vi "Hangup Test.vi"(6 "Aktion Hangup Test":T1, 8 "Status":string, 9 "FID":sgl caption="ppm" format="%.1f") -> (0 "Status":string, 1 "Test beendet?":bool, 2 "countdonw":dbl, 4 "Aktion Hangup Test 2":T1)   [LabVIEW 2020, in "Hangup Check.lvlib"]
uses:
  Hangup Check.lvlib
  Aktion Hangup Test.ctl
  Amium PNS/Aktion FGV Amium Daten.ctl
  AktionFGV Hangup.ctl
  Seiten/CalGas Aufschaltung/FGV CalGas Aktionen.ctl
  Seiten/CalGas Aufschaltung/Auswahl Analysator.ctl
  Analysator Definition/FGV Analysator Definition Aktionen.ctl
  Sprachverwaltung/FGV Aktion Tabelle zerlegen.ctl
  Funktionstasten/Funktionstasten-Aktion.ctl
  Funktionstasten/Zustaende.ctl
  Messdaten/Gewichtung (Stichprobe).ctl
  Seiten/CalGas Aufschaltung/CalGas Aufschaltung.lvlib
  Seiten/FT-IR/FT-IR.lvlib
  Sprachverwaltung/Sprachverwaltung.lvlib
  Funktionstasten/Funktionstasten.lvlib
  Analysator Definition/Analysator Definition.lvlib
  Seiten/FT-IR/FGV FT-IR Aktionen.ctl
  Messdaten/Messdaten.lvlib
  Messdaten/Aktionen FGV Messdaten.ctl
  Amium PNS/Amium PNS.lvlib
  Linearisierung V2/Linearisierung v2.lvlib
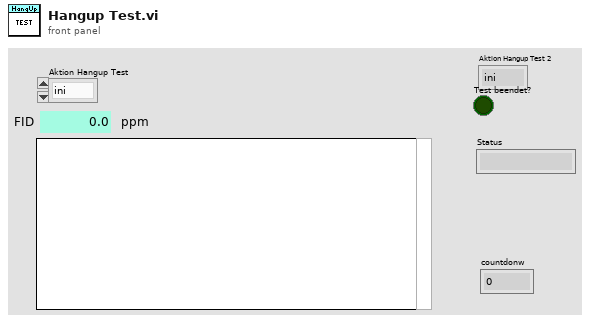
[diagram p1: front panel]
types:
  T1 = typedef "Hangup Check.lvlib/Aktion Hangup Test.ctl" = enum16{"ini", "0-Gas aufschalten", "warten", "E-Gas aufschalten", "auswerten", "Fertig"}
  T2 = typedef "Amium PNS.lvlib/Aktion FGV Amium Daten.ctl" = enum16{"lesen", "Komm Daten", "Daten", "Error", "Regler", "Grenzwerte", "laden", "speichern"}
  T3 = typedef "Sprachverwaltung.lvlib/FGV Aktion Tabelle zerlegen.ctl" = enum16{"laden", "vereinzeln", "speichern"}
  T4 = typedef "Analysator Definition.lvlib/FGV Analysator Definition Aktionen.ctl" = enum16{"lesen", "MB setzen", "MB KAL setzen", "laden"}
  T5 = typedef "CalGas Aufschaltung.lvlib/Auswahl Analysator.ctl" = enum16{"FT-IR", "FID", "PMA", "PMA/FID/FT-IR"}
  T6 = typedef "CalGas Aufschaltung.lvlib/FGV CalGas Aktionen.ctl" = enum16{"lesen", "Analysator Auswahl", "Def.CalGas", "Aufschaltung CalGas", "laden", "speichern", "KAL extrahieren"}
  T7 = typedef "Hangup Check.lvlib/AktionFGV Hangup.ctl" = enum16{"lesen", "Hangup Settings", "Protokoll", "Pfad", "laden", "speichern"}
  T8 = typedef "Funktionstasten.lvlib/Zustaende.ctl" = enum16{"Standby", "Pause", "Eco", "Messen", "Kalibrieren", "Spülen Filter", "Spülen Leitung", "Umgebungsluft", "0-Gas", "Cal-Gas", "CG zu PNS", "-------------", "Init 1", "Init 2", "Init 3", "Init 4", "Messen vorbereiten", "Messen durchführen", "Exit"}
  T9 = typedef "Funktionstasten.lvlib/Funktionstasten-Aktion.ctl" = enum16{"Initialisieren", "Zustand setzen", "Taste gedrückt", "Fehler speichern", "Lesen", "Manuell", "Remote", "Bitparallel", "Samplepoint", "Zeit Prüfen", "reset Umschalten"}
  T10 = typedef "Messdaten.lvlib/Aktionen FGV Messdaten.ctl" = enum16{"lesen", "schreiben", "löschen", "Mittelwerte", "Komponente"}
  T11 = typedef "Messdaten.lvlib/Gewichtung (Stichprobe).ctl" = enum16{"Sample", "Population"}
  T12 = typedef "FT-IR.lvlib/FGV FT-IR Aktionen.ctl" = enum16{"lesen", "NOG setzen", "NOS setzen", "Initialisieren", "speichern", "ALLES setzen", "FT-IR Spektrum loggen", "Komm Stoppen", "Spektrum LogKonfig"}
  T13 = typedef "Amium PNS.lvlib/Daten Cluster.ctl" = cluster{"Amium Zustände":T14, "Samplepoint am PNS":i16, "Gerätekennung":string, "aktiver Samplepoint":i16[], "Messgasdruck":sgl}
  T14 = typedef "Amium PNS.lvlib/Amium Zustand.ctl" = u16
  T15 = typedef "Hangup Check.lvlib/HangupSettings.ctl" = cluster{"Kalibriergas":T16, "Aufschaltpunkt":T16, "Spangas Aufschaltzeit:":sgl, "Nullgas Aufschaltzeit:":sgl, "Datenerfassungszeit:":sgl, "Grenzwert manuell:":sgl, "Grenzwert:":sgl, "Grenze":T16, "Messbereich":T16, "Spankonzentration [ppm]":sgl, "Grenzwert: C1":sgl}
  T16 = typedef "Auswahlfeld.ctl" = u16
  T17 = typedef "Analysator Definition.lvlib/Betriebsdaten Komponente.ctl" = cluster{"Namen":string[], "MB Namen":string[], "Einheit":string, "MB Aktuell":u16, "MB Endwert":u16, "CalGase":u16[], "MB für KAL":u16[], "CG für KAL":u16[]}
  T18 = typedef "CalGas Aufschaltung.lvlib/Aufschaltung CalGas.ctl" = cluster{"Kalibriergas":T16, "Aufschaltpunkt":T19, "Analysator":T5}
  T19 = typedef "CalGas Aufschaltung.lvlib/Auswahl Aufschaltpunkt.ctl" = enum16{"über Filterblock", "Analysator direkt", "über PNS", "Entnahme", "Gasdivider"}
  T20 = typedef "Zahlen-Eingabefeld.ctl" = sgl
  T21 = typedef "Hangup Check.lvlib/Protokoll.ctl" = cluster{"FID Mittelwert 0":sgl, "FID Mittelwert E":sgl, "Messgasdruck Amium":sgl, "Startzeit":timestamp, "Endzeit":timestamp, "Bestanden?":bool}
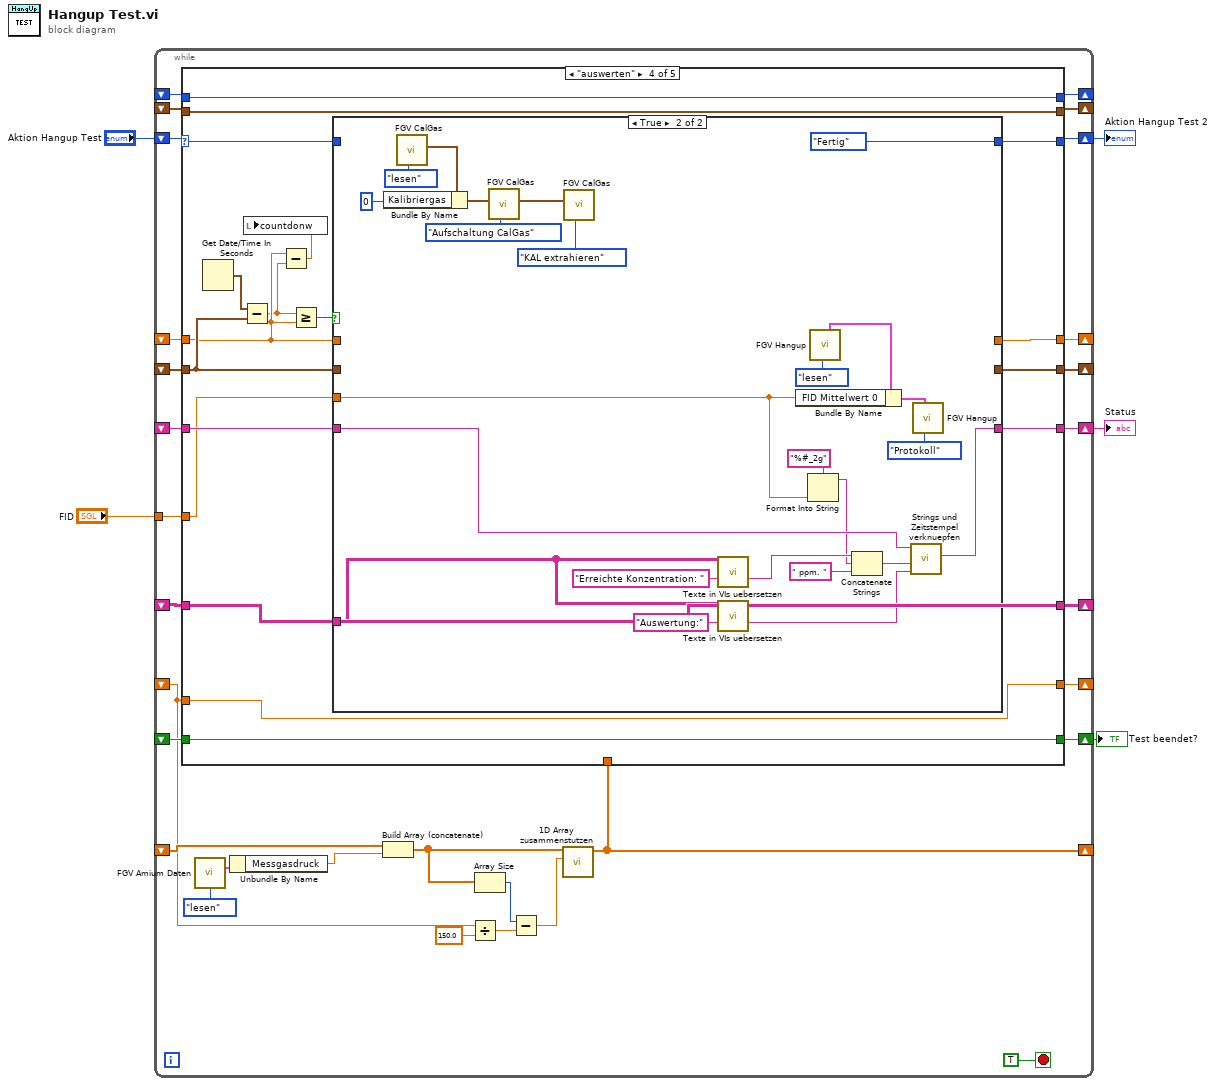
[diagram p0: block diagram]
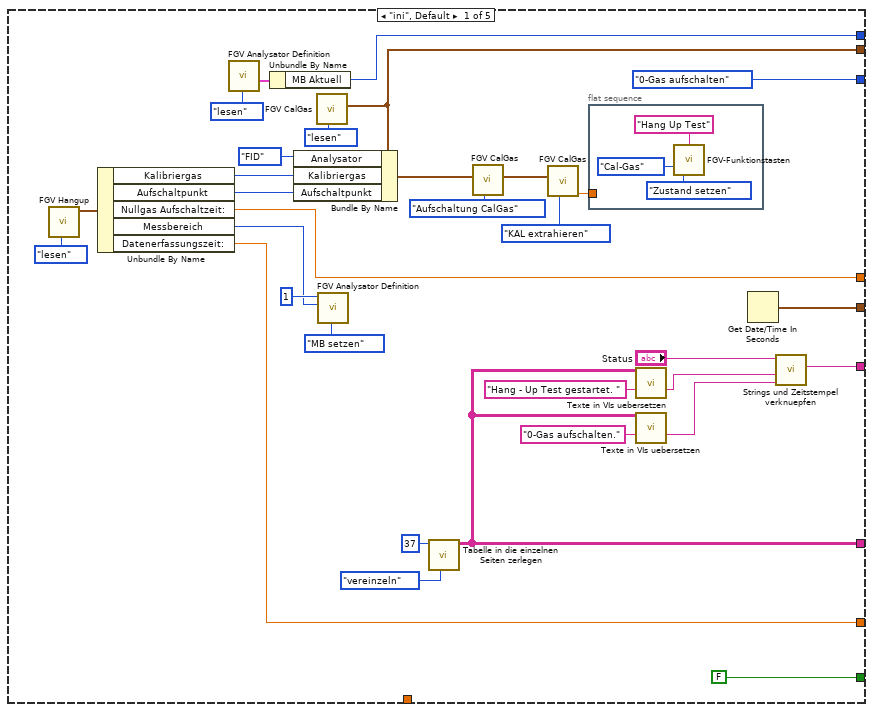
[diagram p2: hidden frame]
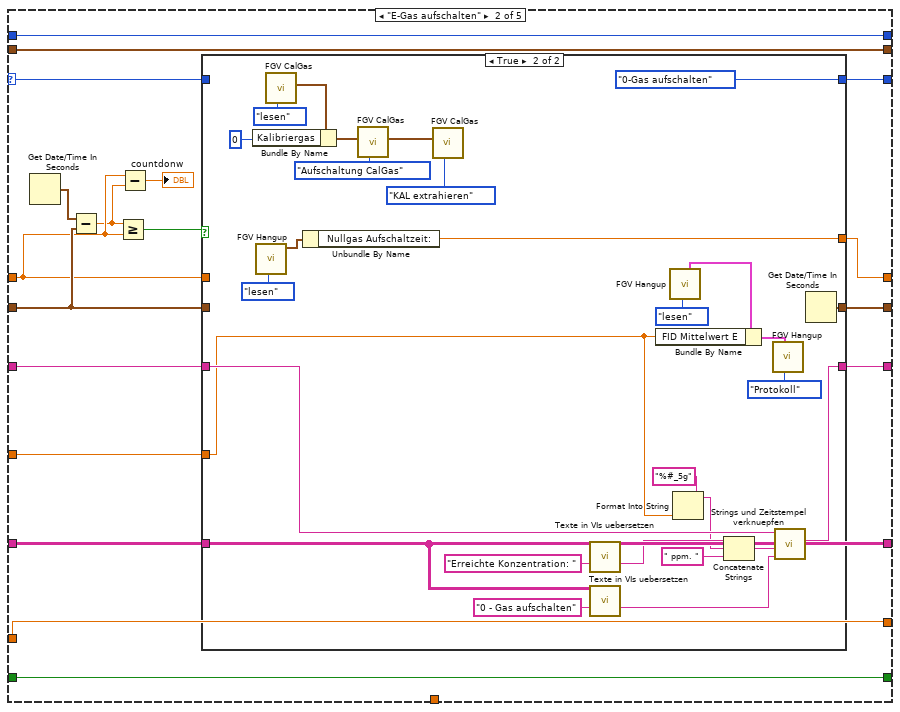
[diagram p3: hidden frame]
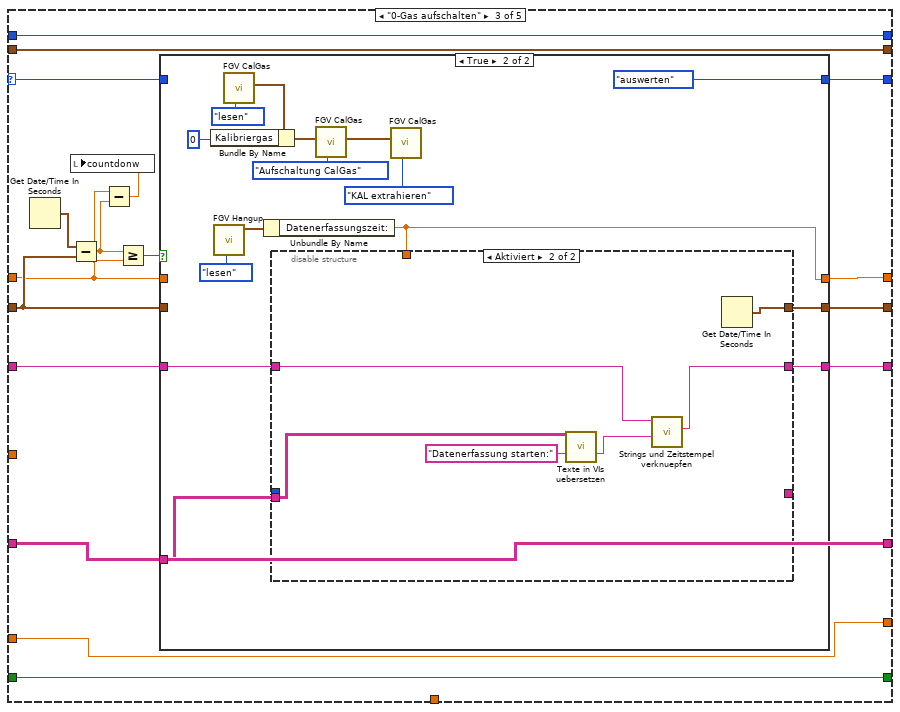
[diagram p5: hidden frame]
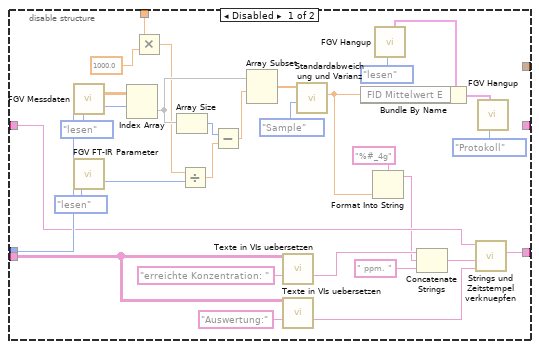
[diagram p7: hidden frame]
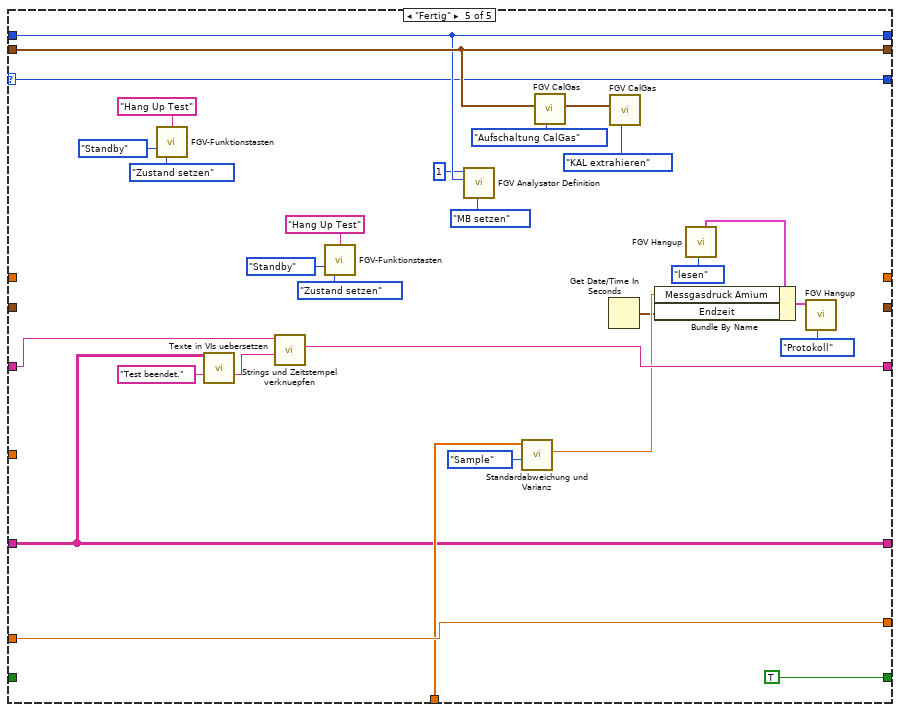
[diagram p9: hidden frame]
diagram:
  n1 = while {
    shift-right: [w34] -> _
    shift-left: _ -> [w33]
    shift-right: [w32] -> w4
    shift-left: _ -> [w31]
    shift-right: [w30] -> _
    shift-left: _ -> [w29]
    shift-right: [w28] -> _
    shift-left: _ -> [w27]
    shift-right: [w26] -> w3
    shift-left: "Aktion Hangup Test" -> [w25]
    shift-right: [w24] -> _
    shift-left: _ -> [w23]
    shift-right: [w22] -> w2
    shift-left: _ -> [w21]
    shift-right: [w9] -> _
    shift-left: _ -> [w18]
    shift-right: [w11] -> _
    shift-left: _ -> [w10]
    shift-right: [w8] -> _
    shift-left: _ -> [w7]
    tunnel: "FID" -> [w6]
    stop <- TRUE stop-if-true
    n2 = call "FGV Amium Daten.vi"("Aktion"=Aktion_FGV_Amium_Daten."lesen") -> ("Amium Daten"=w20:T13)  [unwired: 9 in, 5 out]
    n3 = Unbundle By Name(w20) -> ("Messgasdruck"=w17:sgl)
    n4 = Build Array (concatenate)(w18, w17) -> (w14:sgl[])
    n5 = Divide(x=w10, y=sgl 150.0) -> (x/y=w15:sgl)
    n6 = Array Size(array=w14) -> (size(s)=w16:i32)
    n7 = Subtract(x=w16, y=w15) -> (x-y=w12:sgl)
    n8 = call "1D Array zusammenstutzen.vi"("Anzahl Elemente"=w12, "Messdaten"=w14) -> ("Messdaten"=w9:sgl[])  [unwired: 8 in, 1 out]
    n9 = case shown="\"auswerten\"" w25 {
      selector: w25 -> [_ w85 w134 w207 w250]
      tunnel: [w58 w88 w137 w210 w263] -> w34
      tunnel: w33 -> [_ w88 w137 w210 w263]
      tunnel: [w54 w81 w130 w203 w251] -> w32
      tunnel: w31 -> [_ w82 w131 w204 w252]
      tunnel: [w50 w79 w128 w201 _] -> w30
      tunnel: w29 -> [_ w78 w129 w202 _]
      tunnel: [w49 w80 w127 w200 _] -> w28
      tunnel: w27 -> [_ w74 w123 w196 _]
      tunnel: [Aktion_Hangup_Test."0-Gas aufschalten" ("Aktion Hangup Test") w84 w133 w206 w250] -> w26
      tunnel: [w42 w83 w132 w205 w261] -> w24
      tunnel: w23 -> [_ w83 w132 w205 w261]
      tunnel: [FALSE w77 w126 w199 TRUE] -> w22
      tunnel: w21 -> [_ w77 w126 w199 _]
      tunnel: [w39 w76 w125 w198 w256] -> w11
      tunnel: w10 -> [_ w76 w125 w198 w256]
      tunnel: w9 -> [_ _ _ _ w255]
      tunnel: [w36 w75 w124 w197 w249] -> w8
      tunnel: w7 -> [_ w75 w124 w197 w249]
      tunnel: w6 -> [_ w71 _ w193 _]
      frame "ini", Default {
        n10 = call "FGV Hangup.vi"("Aktion"=AktionFGV_Hangup."lesen") -> ("Hangup Settings"=w66:T15)  [unwired: 6 in, 4 out]
        n11 = Unbundle By Name(w66) -> ("Kalibriergas"=w51:T16, "Aufschaltpunkt"=w59:T16, "Nullgas Aufschaltzeit:"=w49:sgl, "Messbereich"=w41:T16, "Datenerfassungszeit:"=w39:sgl)
        n12 = call "FGV Analysator Definition.vi"("Aktionen"=FGV_Analysator_Definition_Aktionen."lesen") -> ("Betriebsdaten Komponente"=w43:T17)  [unwired: 6 in, 4 out]
        n13 = Unbundle By Name(w43) -> ("MB Aktuell"=w42:u16)
        n14 = call "FGV CalGas.vi"("Aktionen"=FGV_CalGas_Aktionen."lesen") -> ("Aufschaltung CalGas"=w58:T18)  [unwired: 6 in, 4 out]
        n15 = Bundle By Name(cluster=w58, "Analysator"=Auswahl_Analysator."FID", "Kalibriergas"=w51, "Aufschaltpunkt"=w59) -> (w65:T18)
        n16 = call "FGV Analysator Definition.vi"("Aktionen"=FGV_Analysator_Definition_Aktionen."MB setzen", "Messbereich"=w41, "Komponente"=1) -> ()  [unwired: 4 in, 5 out]
        n17 = call "Tabelle in die einzelnen Seiten zerlegen.vi"("Aktion"=FGV_Aktion_Tabelle_zerlegen."vereinzeln", "Index (Seite)"=37) -> ("Sprachliste"=w36:string[][])  [unwired: 7 in, 2 out]
        n18 = call "FGV CalGas.vi"("Aktionen"=FGV_CalGas_Aktionen."Aufschaltung CalGas", "Aufschaltung CalGas"=w65) -> ("Aufschaltung CalGas"=w62:T18)  [unwired: 5 in, 4 out]
        n19 = call "FGV CalGas.vi"("Aktionen"=FGV_CalGas_Aktionen."KAL extrahieren", "Aufschaltung CalGas"=w62) -> ("Konzentration 2"=w48:T20)  [unwired: 5 in, 4 out]
        n20 = flat-sequence {
          tunnel: w48 -> [_]
          frame #0 {
            n21 = call "FGV-Funktionstasten.vi"("Herkunft"="Hang Up Test", "Zustand"=Zustaende."Cal-Gas", "Aktion"=Funktionstasten-Aktion."Zustand setzen") -> ()  [unwired: 5 in, 8 out]
          }
        }
        n22 = call "Texte in VIs uebersetzen.vi"("Sprachliste"=w36, "String zum Übersetzen"="Hang - Up Test gestartet. ") -> ("String zum Übersetzen"=w56:string)  [unwired: 9 in, 4 out]
        n23 = call "Texte in VIs uebersetzen.vi"("Sprachliste"=w36, "String zum Übersetzen"="0-Gas aufschalten.") -> ("String zum Übersetzen"=w53:string)  [unwired: 9 in, 4 out]
        n24 = Get Date/Time In Seconds() -> (seconds since 1Jan1904=w50:timestamp)
        n25 = call "Strings und Zeitstempel verknuepfen.vi"("String 2 hinzufügen"=w53, "String 1 hinzufügen"=w56, "Eingagns String"="Status") -> ("Verknüpfter String"=w54:string)  [unwired: 8 in]
      }
      frame "E-Gas aufschalten" {
        n26 = Get Date/Time In Seconds() -> (seconds since 1Jan1904=w87:timestamp)
        n27 = Subtract(x=w87, y=w78) -> (x-y=w73:dbl)
        n28 = Greater Or Equal?(x=w73, y=w74) -> (x >= y?=w86:bool)
        n29 = Subtract(x=w74, y=w73) -> (x-y=→"countdonw":dbl)
        n30 = case shown="True" w86 {
          tunnel: w85 -> [w92 _]
          tunnel: [w92 Aktion_Hangup_Test."0-Gas aufschalten" ("Aktion Hangup Test")] -> w84
          tunnel: w82 -> [w91 w109]
          tunnel: [w91 w108] -> w81
          tunnel: [w89 w107] -> w80
          tunnel: [w90 w106] -> w79
          tunnel: w78 -> [w90 _]
          tunnel: w74 -> [w89 _]
          tunnel: w75 -> [_ w98]
          tunnel: w71 -> [_ w93]
          frame False {
          }
          frame True {
            n31 = call "FGV Hangup.vi"("Aktion"=AktionFGV_Hangup."lesen") -> ("Hangup Settings"=w112:T15)  [unwired: 6 in, 4 out]
            n32 = call "FGV CalGas.vi"("Aktionen"=FGV_CalGas_Aktionen."lesen") -> ("Aufschaltung CalGas"=w114:T18)  [unwired: 6 in, 4 out]
            n33 = Bundle By Name(cluster=w114, "Kalibriergas"=0) -> (w119:T18)
            n34 = Unbundle By Name(w112) -> ("Nullgas Aufschaltzeit:"=w107:sgl)
            n35 = call "FGV CalGas.vi"("Aktionen"=FGV_CalGas_Aktionen."Aufschaltung CalGas", "Aufschaltung CalGas"=w119) -> ("Aufschaltung CalGas"=w116:T18)  [unwired: 5 in, 4 out]
            n36 = call "FGV CalGas.vi"("Aktionen"=FGV_CalGas_Aktionen."KAL extrahieren", "Aufschaltung CalGas"=w116) -> ()  [unwired: 5 in, 5 out]
            n37 = call "Texte in VIs uebersetzen.vi"("Sprachliste"=w98, "String zum Übersetzen"="Erreichte Konzentration: ") -> ("String zum Übersetzen"=w102:string)  [unwired: 9 in, 4 out]
            n38 = call "Texte in VIs uebersetzen.vi"("Sprachliste"=w98, "String zum Übersetzen"="0 - Gas aufschalten") -> ("String zum Übersetzen"=w104:string)  [unwired: 9 in, 4 out]
            n39 = call "FGV Hangup.vi"("Aktion"=AktionFGV_Hangup."lesen") -> ("Protokoll"=w95:T21)  [unwired: 6 in, 4 out]
            n40 = Bundle By Name(cluster=w95, "FID Mittelwert E"=w93) -> (w97:T21)
            n41 = Format Into String(format string="%#_5g" ("Format-String"), w93) -> (resulting string=w101:string)  [unwired: 2 in, 1 out]
            n42 = Concatenate Strings(w102, w101, " ppm. " ("String")) -> (w99:string)
            n43 = call "FGV Hangup.vi"("Aktion"=AktionFGV_Hangup."Protokoll", "Protokoll"=w97) -> ()  [unwired: 5 in, 5 out]
            n44 = call "Strings und Zeitstempel verknuepfen.vi"("String 2 hinzufügen"=w104, "String 1 hinzufügen"=w99, "Eingagns String"=w109) -> ("Verknüpfter String"=w108:string)  [unwired: 8 in]
            n45 = Get Date/Time In Seconds() -> (seconds since 1Jan1904=w106:timestamp)
          }
        }
      }
      frame "0-Gas aufschalten" {
        n46 = Get Date/Time In Seconds() -> (seconds since 1Jan1904=w136:timestamp)
        n47 = Subtract(x=w136, y=w129) -> (x-y=w122:dbl)
        n48 = Subtract(x=w123, y=w122) -> (x-y=w121:dbl)
        n49 = local write "countdonw"(w121) -> ()
        n50 = Greater Or Equal?(x=w122, y=w123) -> (x >= y?=w135:bool)
        n51 = case shown="True" w135 {
          tunnel: w134 -> [w141 _]
          tunnel: [w141 Aktion_Hangup_Test."auswerten" ("Aktion Hangup Test")] -> w133
          tunnel: w131 -> [w140 w146]
          tunnel: [w140 w143] -> w130
          tunnel: w129 -> [w139 _]
          tunnel: [w139 w142] -> w128
          tunnel: [w138 w144] -> w127
          tunnel: w123 -> [w138 _]
          tunnel: w124 -> [_ w145]
          frame False {
          }
          frame True {
            n52 = call "FGV Hangup.vi"("Aktion"=AktionFGV_Hangup."lesen") -> ("Hangup Settings"=w148:T15)  [unwired: 6 in, 4 out]
            n53 = call "FGV CalGas.vi"("Aktionen"=FGV_CalGas_Aktionen."lesen") -> ("Aufschaltung CalGas"=w150:T18)  [unwired: 6 in, 4 out]
            n54 = Bundle By Name(cluster=w150, "Kalibriergas"=0) -> (w155:T18)
            n55 = Unbundle By Name(w148) -> ("Datenerfassungszeit:"=w144:sgl)
            n56 = disable-structure shown="Aktiviert" {
              disable-tunnel: _ -> [w174 _]
              disable-tunnel: [w169 _] -> _
              disable-tunnel: w146 -> [w168 w191]
              disable-tunnel: w145 -> [w163 w188]
              disable-tunnel: w144 -> [w157 _]
              disable-tunnel: [_ w190] -> w143
              disable-tunnel: [_ w187] -> w142
              frame Disabled {
                n57 = call "FGV Messdaten.vi"("Aktionen"=Aktionen_FGV_Messdaten."lesen") -> ("Messdaten"=w177:sgl[][])  [unwired: 6 in, 8 out]
                n58 = call "FGV FT-IR Parameter.vi"("Aktion"=FGV_FT-IR_Aktionen."lesen") -> ("Zykluszeit Messdatenverteiler"=w186:u32)  [unwired: 11 in, 7 out]
                n59 = Index Array(array=w177, index (row)=w174) -> (element=w178:sgl[])  [unwired: 1 in]
                n60 = Multiply(x=w157, y=sgl 1000.0) -> (x*y=w175:sgl)
                n61 = Array Size(array=w178) -> (size(s)=w181:i32)
                n62 = Divide(x=w175, y=w186) -> (x/y=w180:sgl)
                n63 = Subtract(x=w181, y=w180) -> (x-y=w182:sgl)
                n64 = Array Subset(array=w178, index=w182) -> (w179:sgl[])  [unwired: 1 in]
                n65 = call "Texte in VIs uebersetzen.vi"("Sprachliste"=w163, "String zum Übersetzen"="erreichte Konzentration: ") -> ("String zum Übersetzen"=w172:string)  [unwired: 9 in, 4 out]
                n66 = call "Texte in VIs uebersetzen.vi"("Sprachliste"=w163, "String zum Übersetzen"="Auswertung:") -> ("String zum Übersetzen"=w173:string)  [unwired: 9 in, 4 out]
                n67 = call "Standardabweichung und Varianz.vi"("Gewichtung (Stichprobe)"=Gewichtung_(Stichprobe)."Sample", "X"=w179) -> ("Mittelwert"=w158:sgl)  [unwired: 7 in, 2 out]
                n68 = Format Into String(format string="%#_4g" ("Format-String"), w158) -> (resulting string=w164:string)  [unwired: 2 in, 1 out]
                n69 = call "FGV Hangup.vi"("Aktion"=AktionFGV_Hangup."lesen") -> ("Protokoll"=w160:T21)  [unwired: 6 in, 4 out]
                n70 = Bundle By Name(cluster=w160, "FID Mittelwert E"=w158) -> (w162:T21)
                n71 = Concatenate Strings(w172, w164, " ppm. " ("String")) -> (w170:string)
                n72 = call "Strings und Zeitstempel verknuepfen.vi"("String 2 hinzufügen"=w173, "String 1 hinzufügen"=w170, "Eingagns String"=w168) -> ("Verknüpfter String"=w169:string)  [unwired: 8 in]
                n73 = call "FGV Hangup.vi"("Aktion"=AktionFGV_Hangup."Protokoll", "Protokoll"=w162) -> ()  [unwired: 5 in, 5 out]
              }
              frame Enabled {
                n74 = call "Texte in VIs uebersetzen.vi"("Sprachliste"=w188, "String zum Übersetzen"="Datenerfassung starten:") -> ("String zum Übersetzen"=w189:string)  [unwired: 9 in, 4 out]
                n75 = call "Strings und Zeitstempel verknuepfen.vi"("String 1 hinzufügen"=w189, "Eingagns String"=w191) -> ("Verknüpfter String"=w190:string)  [unwired: 9 in]
                n76 = Get Date/Time In Seconds() -> (seconds since 1Jan1904=w187:timestamp)
              }
            }
            n77 = call "FGV CalGas.vi"("Aktionen"=FGV_CalGas_Aktionen."Aufschaltung CalGas", "Aufschaltung CalGas"=w155) -> ("Aufschaltung CalGas"=w152:T18)  [unwired: 5 in, 4 out]
            n78 = call "FGV CalGas.vi"("Aktionen"=FGV_CalGas_Aktionen."KAL extrahieren", "Aufschaltung CalGas"=w152) -> ()  [unwired: 5 in, 5 out]
          }
        }
      }
      frame "auswerten" {
        n79 = Get Date/Time In Seconds() -> (seconds since 1Jan1904=w209:timestamp)
        n80 = Subtract(x=w209, y=w202) -> (x-y=w195:dbl)
        n81 = Subtract(x=w196, y=w195) -> (x-y=w194:dbl)
        n82 = local write "countdonw"(w194) -> ()
        n83 = Greater Or Equal?(x=w195, y=w196) -> (x >= y?=w208:bool)
        n84 = case shown="True" w208 {
          tunnel: w207 -> [w214 _]
          tunnel: [w214 Aktion_Hangup_Test."Fertig" ("Aktion Hangup Test")] -> w206
          tunnel: w204 -> [w213 w225]
          tunnel: [w213 w226] -> w203
          tunnel: w202 -> [w212 _]
          tunnel: [w212 _] -> w201
          tunnel: [w211 _] -> w200
          tunnel: w196 -> [w211 _]
          tunnel: w197 -> [_ w220]
          tunnel: w193 -> [_ w215]
          frame False {
          }
          frame True {
            n85 = call "FGV CalGas.vi"("Aktionen"=FGV_CalGas_Aktionen."lesen") -> ("Aufschaltung CalGas"=w232:T18)  [unwired: 6 in, 4 out]
            n86 = Bundle By Name(cluster=w232, "Kalibriergas"=0) -> (w237:T18)
            n87 = call "FGV CalGas.vi"("Aktionen"=FGV_CalGas_Aktionen."Aufschaltung CalGas", "Aufschaltung CalGas"=w237) -> ("Aufschaltung CalGas"=w234:T18)  [unwired: 5 in, 4 out]
            n88 = call "FGV CalGas.vi"("Aktionen"=FGV_CalGas_Aktionen."KAL extrahieren", "Aufschaltung CalGas"=w234) -> ()  [unwired: 5 in, 5 out]
            n89 = call "Texte in VIs uebersetzen.vi"("Sprachliste"=w220, "String zum Übersetzen"="Erreichte Konzentration: ") -> ("String zum Übersetzen"=w229:string)  [unwired: 9 in, 4 out]
            n90 = call "Texte in VIs uebersetzen.vi"("Sprachliste"=w220, "String zum Übersetzen"="Auswertung:") -> ("String zum Übersetzen"=w230:string)  [unwired: 9 in, 4 out]
            n91 = Format Into String(format string="%#_2g" ("Format-String"), w215) -> (resulting string=w221:string)  [unwired: 2 in, 1 out]
            n92 = call "FGV Hangup.vi"("Aktion"=AktionFGV_Hangup."lesen") -> ("Protokoll"=w217:T21)  [unwired: 6 in, 4 out]
            n93 = Bundle By Name(cluster=w217, "FID Mittelwert 0"=w215) -> (w219:T21)
            n94 = Concatenate Strings(w229, w221, " ppm. " ("String")) -> (w227:string)
            n95 = call "Strings und Zeitstempel verknuepfen.vi"("String 2 hinzufügen"=w230, "String 1 hinzufügen"=w227, "Eingagns String"=w225) -> ("Verknüpfter String"=w226:string)  [unwired: 8 in]
            n96 = call "FGV Hangup.vi"("Aktion"=AktionFGV_Hangup."Protokoll", "Protokoll"=w219) -> ()  [unwired: 5 in, 5 out]
          }
        }
      }
      frame "Fertig" {
        n97 = call "FGV-Funktionstasten.vi"("Herkunft"="Hang Up Test", "Zustand"=Zustaende."Standby", "Aktion"=Funktionstasten-Aktion."Zustand setzen") -> ()  [unwired: 5 in, 8 out]
        n98 = call "Texte in VIs uebersetzen.vi"("Sprachliste"=w249, "String zum Übersetzen"="Test beendet.") -> ("String zum Übersetzen"=w254:string)  [unwired: 9 in, 4 out]
        n99 = call "Strings und Zeitstempel verknuepfen.vi"("String 1 hinzufügen"=w254, "Eingagns String"=w252) -> ("Verknüpfter String"=w251:string)  [unwired: 9 in]
        n100 = call "FGV-Funktionstasten.vi"("Herkunft"="Hang Up Test", "Zustand"=Zustaende."Standby", "Aktion"=Funktionstasten-Aktion."Zustand setzen") -> ()  [unwired: 5 in, 8 out]
        n101 = call "FGV Analysator Definition.vi"("Aktionen"=FGV_Analysator_Definition_Aktionen."MB setzen", "Messbereich"=w261, "Komponente"=1) -> ()  [unwired: 4 in, 5 out]
        n102 = call "Standardabweichung und Varianz.vi"("Gewichtung (Stichprobe)"=Gewichtung_(Stichprobe)."Sample", "X"=w255) -> ("Mittelwert"=w244:sgl)  [unwired: 7 in, 2 out]
        n103 = call "FGV CalGas.vi"("Aktionen"=FGV_CalGas_Aktionen."Aufschaltung CalGas", "Aufschaltung CalGas"=w263) -> ("Aufschaltung CalGas"=w265:T18)  [unwired: 5 in, 4 out]
        n104 = Get Date/Time In Seconds() -> (seconds since 1Jan1904=w243:timestamp)
        n105 = call "FGV CalGas.vi"("Aktionen"=FGV_CalGas_Aktionen."KAL extrahieren", "Aufschaltung CalGas"=w265) -> ()  [unwired: 5 in, 5 out]
        n106 = call "FGV Hangup.vi"("Aktion"=AktionFGV_Hangup."lesen") -> ("Protokoll"=w246:T21)  [unwired: 6 in, 4 out]
        n107 = Bundle By Name(cluster=w246, "Messgasdruck Amium"=w244, "Endzeit"=w243) -> (w248:T21)
        n108 = call "FGV Hangup.vi"("Aktion"=AktionFGV_Hangup."Protokoll", "Protokoll"=w248) -> ()  [unwired: 5 in, 5 out]
      }
    }
  }
  "Status" <- w4
  "Aktion Hangup Test 2" <- w3
  "Test beendet?" <- w2
